vi "Expand the Compact PDO of RX TX.vi"(6 "Number":u16, 7 "RX?":bool, 8 "error in (no error)":errorcluster, 9 "Existing Indexs":u16[](array[numeric]), 10 "CompactPDO":u8, 11 "Arr Refnum":refnum<vi>) -> (0 "error out":errorcluster)   [LabVIEW 2013]
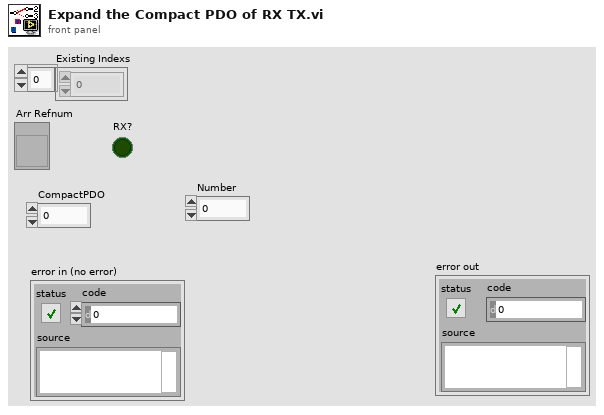
[diagram p1: front panel]
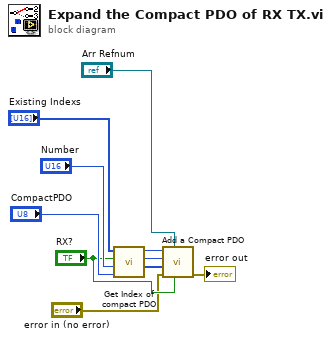
[diagram p0: block diagram]
diagram:
  n1 = call "Get Index of compact PDO.vi"("CompactPDO"="CompactPDO", "Number of PDO"="Number", "RX ?"="RX?", "Existing Indexs"="Existing Indexs") -> ("Index of Compact PDO"=w7:u16[], "Count of Sub Items"=w6:i32, "Start"=w5:u16)  [unwired: 5 in]
  n2 = call "Add a Compact PDO.vi"("RX?"="RX?", "Arr Refnum"="Arr Refnum", "error in (no error)"="error in (no error)", "Index of Compact PDO"=w7, "Count of Sub Items"=w6, "Start"=w5) -> ("error out"=→"error out":errorcluster)  [unwired: 5 in]
